vi "SaveDeviceHeader.vi"(4 "Humidity":dbl, 5 "Array Lengths":i32, 6 "Temperature":dbl, 7 "no. of arrays":i32, 8 "error in (no error)":errorcluster, 9 "Array Titles":string, 10 "Filename":string, 11 "File Refnum in":refnum<file>) -> (0 "error out":errorcluster, 2 "Header string":string, 3 "File Refnum out":refnum<file>)   [LabVIEW 2013]
uses:
  globals/RunInformation.vi
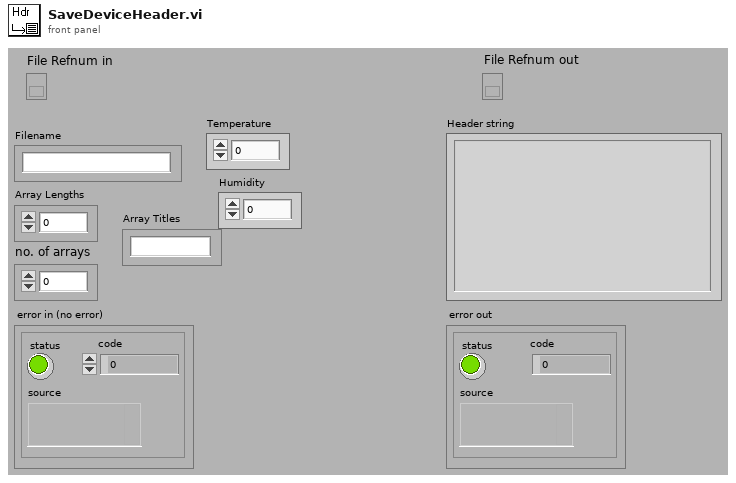
[diagram p1: front panel]
types:
  T1 = cluster{"Institute":string, "Manufacturers":string[], "Devices":string[], "Serialnumbers Lookup DB":string, "Data directory":string, "www directory":string, "List of known users":string[]}
  T2 = cluster{"Sensor Serial No.:":string, "Wafer Serial No.:":string, "Batch:":string, "Manufacturer:":string, "Device Category:":string, "Database Serial No.:":string, "Initiated:":string, "Test":string, "Instruments used:":string, "Probeplan used:":string, "End of Run comment:":string, "User:":string}
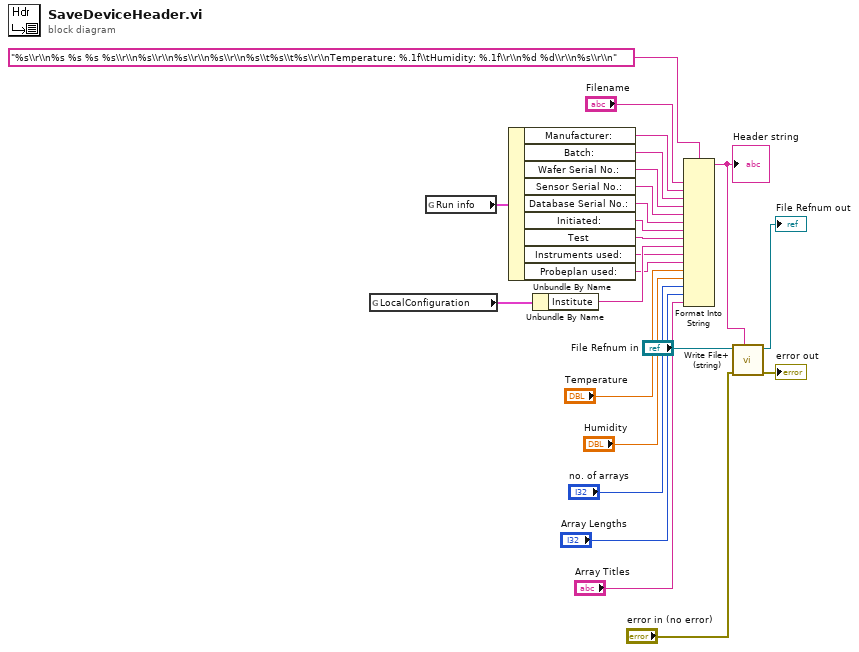
[diagram p0: block diagram]
diagram:
  n1 = global read "RunInformation.vi" "LocalConfiguration"() -> (w13:T1)
  n2 = global read "RunInformation.vi" "Run info"() -> (w24:T2)
  n3 = Unbundle By Name(w24) -> ("Manufacturer:"=w21:string, "Batch:"=w20:string, "Wafer Serial No.:"=w19:string, "Sensor Serial No.:"=w18:string, "Database Serial No.:"=w17:string, "Initiated:"=w16:string, "Test"=w15:string, "Instruments used:"=w11:string, "Probeplan used:"=w10:string)
  n4 = Unbundle By Name(w13) -> ("Institute"=w12:string)
  n5 = Format Into String(format string="%s\\r\\n%s %s %s %s\\r\\n%s\\r\\n%s\\r\\n%s\\r\\n%s\\t%s\\t%s\\r\\nTemperature: %.1f\\tHumidity: %.1f\\r\\n%d %d\\r\\n%s\\r\\n", "Filename", w21, w20, w19, w18, w17, w16, w15, w12, w11, w10, "Temperature", "Humidity", "no. of arrays", "Array Lengths", "Array Titles") -> (resulting string=w14:string)  [unwired: 2 in, 1 out]
  "Header string" <- w14
  n6 = call <vilib>:"Write File+ (string).vi"("string"=w14, "error in (no error)"="error in (no error)", "refnum"="File Refnum in") -> ("error out"=→"error out":errorcluster, "dup refnum"=→"File Refnum out":refnum<file>)  [unwired: 4 in, 1 out]
